vi "Prepare_dataST.vi"(1 "Active Sensors":bool[](array[boolean]), 2 "ranges":bool[](array[boolean]), 3 "Controls[]":refnum<vi>[](array[refnum]), 4 "Flag_215":bool, 5 "error in":errorcluster, 6 "struct":bool, 7 "chkeach_ch":bool, 9 "chk2scan":bool) -> (12 "Meas_rang":i32[](array[numeric]), 13 "Refdata_struct":refnum<k24>[](array[refnum]), 15 "Meas_monitor_struct":refnum<k24>[](array[refnum]), 16 "Data_struct":refnum<k24>[](array[refnum]), 17 "Ref_monitordata_struct":refnum<k24>[](array[refnum]), 18 "Mergedata_struct":refnum<k24>[](array[refnum]), 19 "error out":errorcluster)   [LabVIEW 2017]
doc: "prepare data struct & hold instrument condition"
uses:
  D:/test/PDLSTS/LV_PDL_Sample/DLL/STSProcess.dll
  DLL/STSProcess.dll
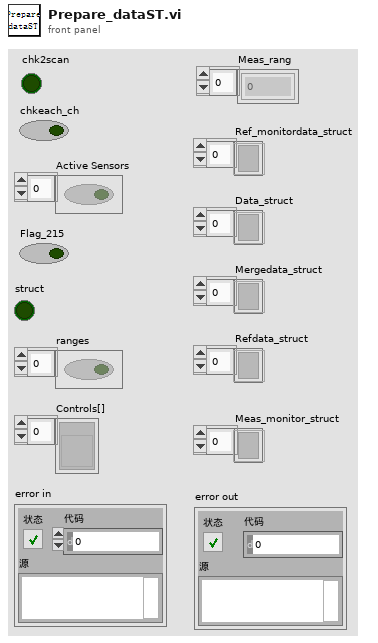
[diagram p1: front panel]
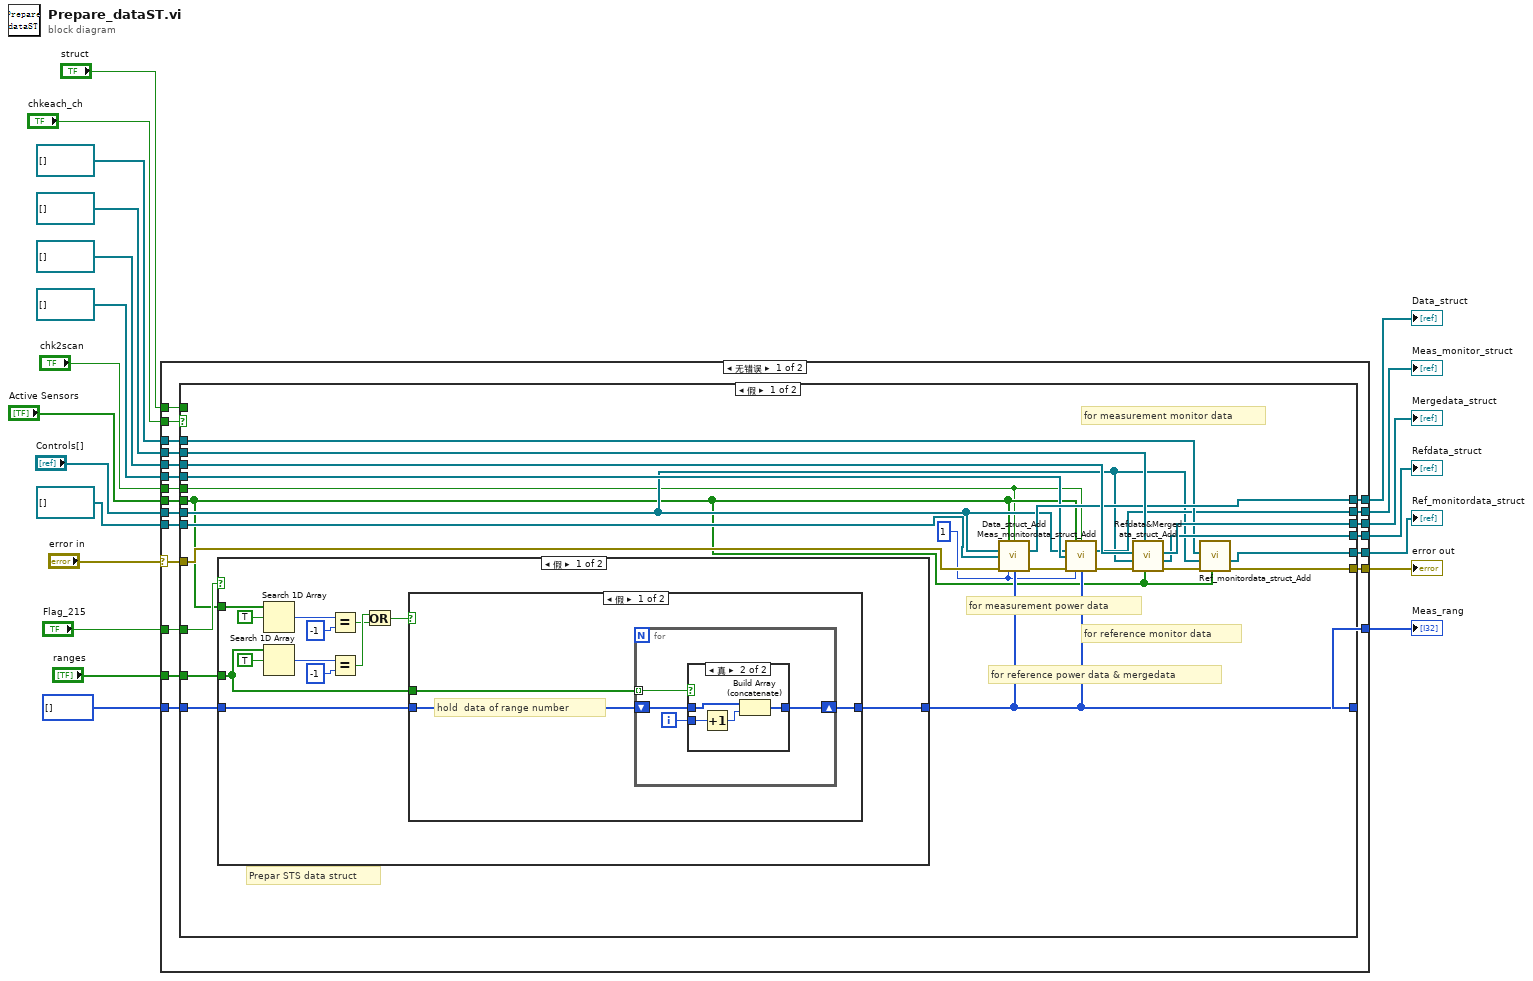
[diagram p0: block diagram]
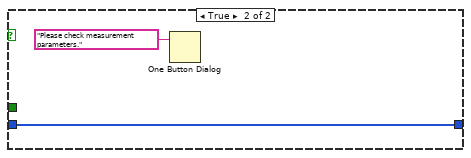
[diagram p3: hidden frame]
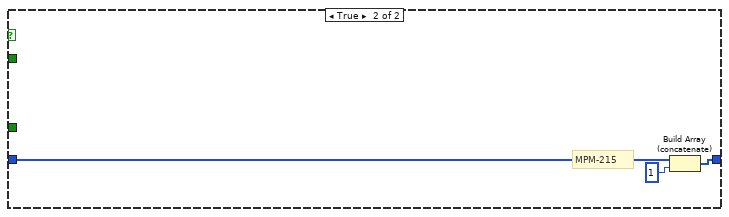
[diagram p4: hidden frame]
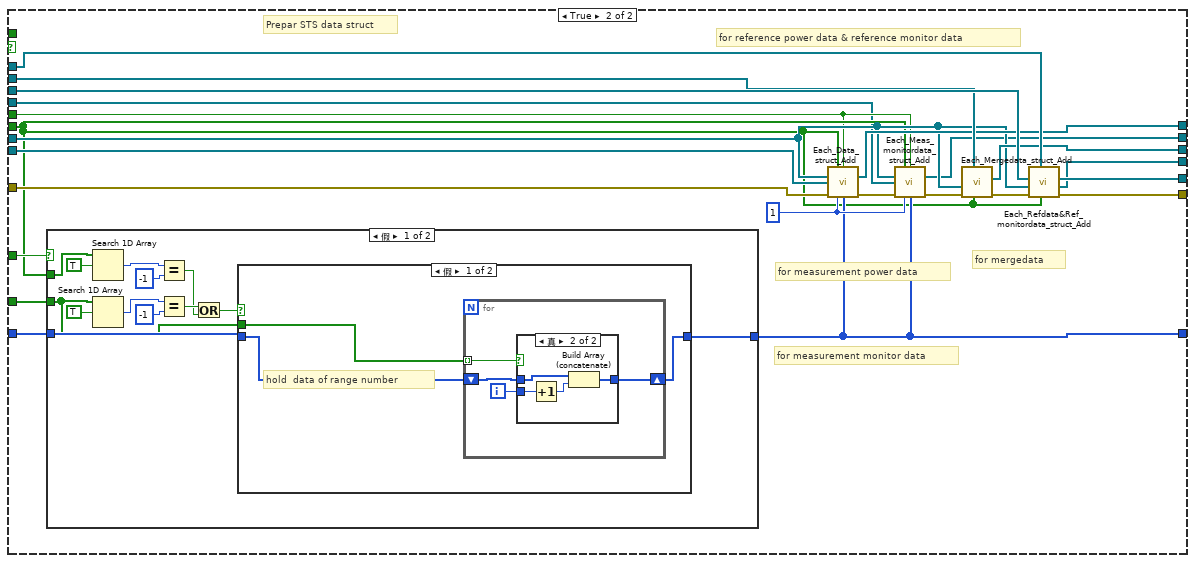
[diagram p5: hidden frame]
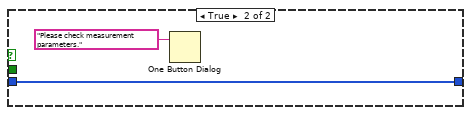
[diagram p7: hidden frame]
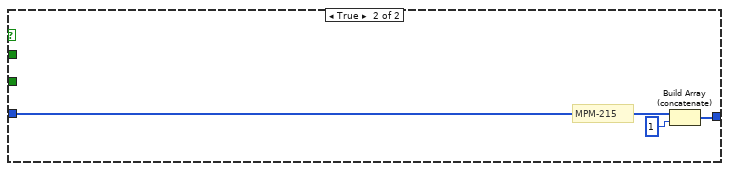
[diagram p8: hidden frame]
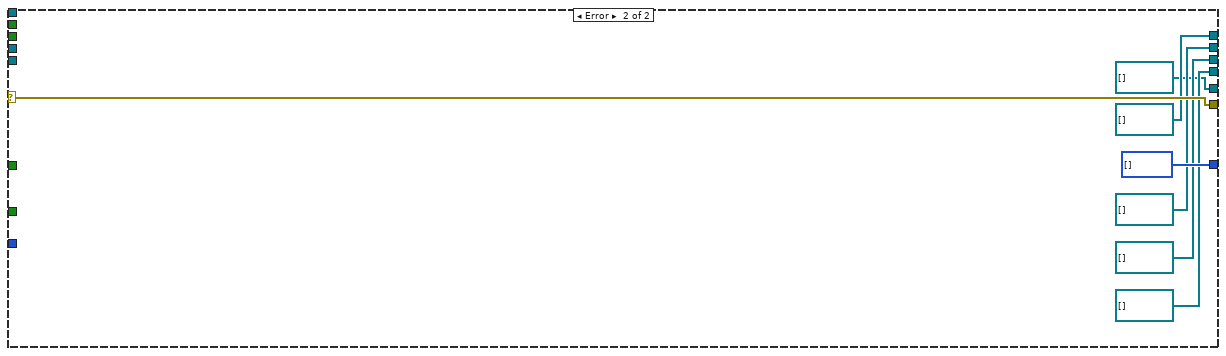
[diagram p9: hidden frame]
diagram:
  n1 = case shown="无错误" "error in" {
    selector: "error in" -> [w23 w155]
    tunnel: "ranges" -> [w42 _]
    tunnel: "Flag_215" -> [w41 _]
    tunnel: "Controls[]" -> [w40 _]
    tunnel: "Active Sensors" -> [w39 _]
    tunnel: "chkeach_ch" -> [w38 _]
    tunnel: "struct" -> [w37 _]
    tunnel: refnum<k24>[] [] ("Data_struct") -> [w36 _]
    tunnel: refnum<k24>[] [] ("Ref_monitordata_struct") -> [w35 _]
    tunnel: refnum<k24>[] [] ("Mergedata_struct") -> [w34 _]
    tunnel: refnum<k24>[] [] ("Meas_monitor_struct") -> [w33 _]
    tunnel: refnum<k24>[] [] ("Refdata_struct") -> [w32 _]
    tunnel: [w31 refnum<k24>[] [] ("Mergedata_struct")] -> w10
    tunnel: [w30 refnum<k24>[] [] ("Data_struct")] -> w9
    tunnel: [w29 refnum<k24>[] [] ("Meas_monitor_struct")] -> w8
    tunnel: [w28 refnum<k24>[] [] ("Refdata_struct")] -> w7
    tunnel: [w27 refnum<k24>[] [] ("Ref_monitordata_struct")] -> w6
    tunnel: i32[] [] ("Meas_rang") -> [w26 _]
    tunnel: [w25 i32[] [] ("Meas_rang")] -> w4
    tunnel: [w24 w155] -> w2
    tunnel: "chk2scan" -> [w22 _]
    frame No Error {
      n2 = case shown="假" w38 {
        tunnel: w39 -> [w45 w100]
        tunnel: w40 -> [w46 w101]
        tunnel: w36 -> [w65 w107]
        tunnel: w33 -> [w50 w97]
        tunnel: w32 -> [w64 w111]
        tunnel: w34 -> [w63 w109]
        tunnel: w35 -> [w54 w113]
        tunnel: w26 -> [w62 w118]
        tunnel: w41 -> [w61 w117]
        tunnel: w42 -> [w60 w116]
        tunnel: w37 -> [_ _]
        tunnel: [w59 w108] -> w31
        tunnel: [w58 w106] -> w30
        tunnel: [w51 w96] -> w29
        tunnel: [w57 w110] -> w28
        tunnel: [w55 w112] -> w27
        tunnel: [w47 w102] -> w25
        tunnel: [w52 w104] -> w24
        tunnel: w23 -> [w56 w115]
        tunnel: w22 -> [w44 w99]
        frame False {
          w43 = 1 ("sweep_count")
          # "for measurement monitor data"
          # "for measurement power data"
          # "for reference power data & mergedata"
          # "for reference monitor data"
          # "Prepar STS data struct"
          n3 = case shown="假" w61 {
            tunnel: w62 -> [w68 w95]
            tunnel: [w67 w93] -> w47
            tunnel: w45 -> [w78 _]
            tunnel: w60 -> [w66 _]
            frame False {
              n4 = Search 1D Array(1D array=w78, element=TRUE ("元素")) -> (index of element=w76:i32)  [unwired: 1 in]
              n5 = Search 1D Array(1D array=w66, element=TRUE ("元素")) -> (index of element=w73:i32)  [unwired: 1 in]
              n6 = Equal?(x=w76, y=-1) -> (x = y?=w70:bool)
              n7 = Equal?(x=w73, y=-1) -> (x = y?=w71:bool)
              n8 = Or(x=w71, y=w70) -> (x .or. y?=w69:bool)
              n9 = case shown="假" w69 {
                tunnel: w66 -> [w81 _]
                tunnel: w68 -> [w80 w91]
                tunnel: [w79 w91] -> w67
                frame False {
                  # "hold  data of range number"
                  n10 = for {
                    tunnel: w81 -> [w85] mode=indexing
                    shift-right: [w82] -> w79
                    shift-left: w80 -> [w84]
                    i -> [w83]
                    n11 = case shown="真" w85 {
                      tunnel: w84 -> [w86 w90]
                      tunnel: w83 -> [_ w88]
                      tunnel: [w86 w87] -> w82
                      frame False {
                      }
                      frame True {
                        n12 = Increment(x=w88) -> (x+1=w89:i32)
                        n13 = Build Array (concatenate)(w90, w89) -> (w87:i32[])
                      }
                    }
                  }
                }
                frame True {
                  n14 = One Button Dialog(message="Please check measurement parameters." ("消息")) -> ()  [unwired: 1 in, 1 out]
                }
              }
            }
            frame True {
              # "MPM-215"
              n15 = Build Array (concatenate)(w95, 1) -> (w93:i32[])
            }
          }
          n16 = call "Data_struct_Add.vi"("Active Sensors"=w45, "chk2scan"=w44, "Controls[]"=w46, "Data_struct输入"=w65, "错误输入（无错误）"=w56, "sweep_count"=w43, "Meas_rang"=w47) -> ("Data_struct输出"=w58:refnum<k24>[], "错误输出"=w49:errorcluster)  [unwired: 7 in]
          n17 = call "Meas_monitordata_struct_Add.vi"("Active Sensors"=w45, "chk2scan"=w44, "Controls[]"=w46, "Meas_monitordata_struct输入"=w50, "错误输入（无错误）"=w49, "sweep_count"=w43, "Meas_rang"=w47) -> ("Meas_monitordata_struct输出"=w51:refnum<k24>[], "错误输出"=w48:errorcluster)  [unwired: 7 in]
          n18 = call "Refdata&Mergedata_struct_Add.vi"("Active Sensors"=w45, "Mergedata_struct输入"=w63, "错误输入（无错误）"=w48, "Controls[]"=w46, "Refdata_struct输入"=w64) -> ("错误输出"=w53:errorcluster, "Refdata_struct输出"=w57:refnum<k24>[], "Mergedata_struct输出"=w59:refnum<k24>[])  [unwired: 4 in]
          n19 = call "Ref_monitordata_struct_Add.vi"("Active Sensors"=w45, "错误输入（无错误）"=w53, "Controls[]"=w46, "Ref_monitordata_struct"=w54) -> ("错误输出"=w52:errorcluster, "Ref_monitordata_struct"=w55:refnum<k24>[])  [unwired: 6 in]
        }
        frame True {
          w105 = 1 ("sweep_count")
          # "for reference power data & reference monitor data"
          # "for mergedata"
          # "for measurement monitor data"
          # "for measurement power data"
          # "Prepar STS data struct"
          n20 = case shown="假" w117 {
            tunnel: w118 -> [w121 w148]
            tunnel: [w120 w146] -> w102
            tunnel: w100 -> [w131 _]
            tunnel: w116 -> [w119 _]
            frame False {
              n21 = Search 1D Array(1D array=w131, element=TRUE ("元素")) -> (index of element=w129:i32)  [unwired: 1 in]
              n22 = Search 1D Array(1D array=w119, element=TRUE ("元素")) -> (index of element=w126:i32)  [unwired: 1 in]
              n23 = Equal?(x=w129, y=-1) -> (x = y?=w123:bool)
              n24 = Equal?(x=w126, y=-1) -> (x = y?=w124:bool)
              n25 = Or(x=w124, y=w123) -> (x .or. y?=w122:bool)
              n26 = case shown="假" w122 {
                tunnel: w119 -> [w134 _]
                tunnel: w121 -> [w133 w144]
                tunnel: [w132 w144] -> w120
                frame False {
                  # "hold  data of range number"
                  n27 = for {
                    tunnel: w134 -> [w138] mode=indexing
                    shift-right: [w135] -> w132
                    shift-left: w133 -> [w137]
                    i -> [w136]
                    n28 = case shown="真" w138 {
                      tunnel: w137 -> [w139 w143]
                      tunnel: w136 -> [_ w141]
                      tunnel: [w139 w140] -> w135
                      frame False {
                      }
                      frame True {
                        n29 = Increment(x=w141) -> (x+1=w142:i32)
                        n30 = Build Array (concatenate)(w143, w142) -> (w140:i32[])
                      }
                    }
                  }
                }
                frame True {
                  n31 = One Button Dialog(message="Please check measurement parameters." ("消息")) -> ()  [unwired: 1 in, 1 out]
                }
              }
            }
            frame True {
              # "MPM-215"
              n32 = Build Array (concatenate)(w148, 1) -> (w146:i32[])
            }
          }
          n33 = call "Each_Data_struct_Add.vi"("Active Sensors"=w100, "chk2scan"=w99, "Controls[]"=w101, "Data_struct输入"=w107, "错误输入（无错误）"=w115, "sweep_count"=w105, "Meas_rang"=w102) -> ("Data_struct输出"=w106:refnum<k24>[], "错误输出"=w103:errorcluster)  [unwired: 7 in]
          n34 = call "Each_Meas_monitordata_struct_Add.vi"("Active Sensors"=w100, "chk2scan"=w99, "Controls[]"=w101, "Meas_monitordata_struct输入"=w97, "错误输入（无错误）"=w103, "sweep_count"=w105, "Meas_rang"=w102) -> ("Meas_monitordata_struct输出"=w96:refnum<k24>[], "错误输出"=w98:errorcluster)  [unwired: 7 in]
          n35 = call "Each_Mergedata_struct_Add.vi"("Active Sensors"=w100, "Mergedata_struct输入"=w109, "错误输入（无错误）"=w98, "Controls[]"=w101) -> ("错误输出"=w114:errorcluster, "Mergedata_struct输出"=w108:refnum<k24>[])  [unwired: 6 in]
          n36 = call "Each_Refdata&Ref_monitordata_struct_Add.vi"("Active Sensors"=w100, "Ref_monitordata_struct输入"=w113, "错误输入（无错误）"=w114, "Controls[]"=w101, "Refdata_struct输入"=w111) -> ("错误输出"=w104:errorcluster, "Refdata_struct输出"=w110:refnum<k24>[], "Ref_monitordata_struct输出"=w112:refnum<k24>[])  [unwired: 4 in]
        }
      }
    }
    frame Error {
    }
  }
  "Ref_monitordata_struct" <- w6
  "Mergedata_struct" <- w10
  "Refdata_struct" <- w7
  "Meas_monitor_struct" <- w8
  "Data_struct" <- w9
  "Meas_rang" <- w4
  "error out" <- w2
